vi "MinimalSynthApp.vi"(0 "Choose Directory":path) -> ()   [LabVIEW 2022 SP3]
uses:
  <vilib>/Analysis/NI_AALBase.lvlib
panel:
  out "Array":i16[][](array[numeric])
  out "x-y":u32
  in  "One Way Receive":bool
  in  "Recip processing":bool
  in  "Recip Processing":u16[][](array[ring])=[[1, 2, 2, 2, 2], [0, 1, 2, 2, 2], [0, 0, 1, 2, 2], [0, 0, 0, 1, 2], [0, 0, 0, 0, 1]] items=["0", "1", "2"]
  in  "Set to Focus":i32=1 min=1 max=5 step=1
  in  "Type of Mean":u16(ring)=3 items=["Mean from lines", "Mean just lines", "Poly Mean", "No mean"]
  in  "Display Plots":bool=TRUE
  in  "Axis scaling":bool=TRUE
  in  "Compress":bool
  in  "Tansducer":u16(ring)=1 items=["F2 40 MHz", "F3 20 MHz"]
  in  "F3 20 MHz":dbl[](array[numeric])=[0.0, 0.0021173000000000003, 0.002217038688303391, 0.003063649156506908, 0.0031631091439381287, 0.0038030513383040436, 0.003902223261134889, 0.004435332245982045, 0.004534208485358321, 0.004999044189180914]
  in  "Round to ROC?":bool=TRUE
  out "ROC (mm)":dbl=0.012
  out "Current File":string
  in  "file ext":string="*1to1*"
  out "zone size mm":dbl format="%#_3g"
  in  "Save Data":bool
  out "c (m/s)":i32=1485
  in  "F2 40MHz":sgl[](array[numeric])=[0.0, 0.00132, 0.00142, 0.0019, 0.002, 0.00236, 0.00245, 0.00275, 0.00285, 0.0031]
  in  "F- zones":i16=41
  out "Focal zones m":sgl[](array[numeric])=[0.0085, 0.009, 0.0095, 0.01, 0.0105, 0.011, 0.0115, 0.012, 0.0125, 0.013, 0.0135, 0.014, 0.0145, 0.015]
  out "Synth Aperture":dbl[][](graph)
  in  "Use Selected Files":bool
  in  "Listbox":i32[](listbox)
  # "Dimension of arrays for processing"
  # "XMT"
  # "RCV"
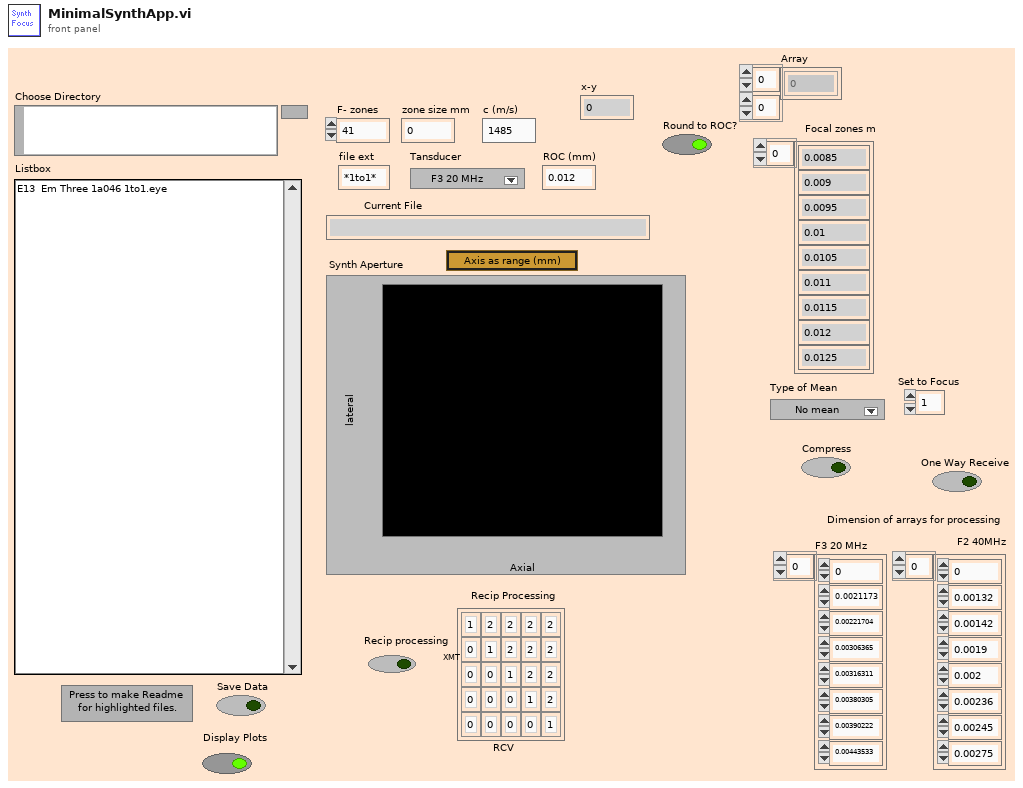
[diagram p1: front panel]
types:
  T1 = typedef "Header.ctl" = cluster{"header info":cluster{"Header":string, "Head length":i16}, "A/D info":cluster{"# rf points per line":u16, "# lines per scan":u16, "sample rate MHz":u16, "# A/D bits":i16, "# bytes per A/D":u16, "TGC Flag":u16, "A/D Type":string}, "Tranducer Info":cluster{"bandwidth":sgl, "center freq":sgl, "start freq":sgl, "ID":i32}, "Scan Info":cluster{"delay":sgl, "pivot distance":sgl, "sector scan angle":sgl, "operator":string, "Scan Mode":string, "location":string}, "Time/Date Info":cluster{"date":string, "time":string}, "RF Info":cluster{"RF file name":string, "RF file att":string, "RF cal file name":string, "RF cal file att":string}, "Patient Info":cluster{"ID":string, "extended ID":string, "age":u16, "sex":string, "previously\nscanned":string, "PSA":sgl, "LOS":u8, "Ethnicty 2":u8, "Race":u8}, "Tissue Type":cluster{"organ":i16, "disease type":i16, "disease location":i16}, "Votage scaling":cluster{"Digitizer (dB)":sgl, "Gain (dB)":sgl, "Atten (dB)":sgl}, "Comment":string, "Misc Info":cluster{"avg num":i16, "c speed":i16, "Div By or SF zones":i16, "XMIT CHS":u8, "RCV CHS":u8}, "Therapy Parameters":cluster{"Theraputic Freq (MHz)":sgl, "Time on (s)":sgl, "Therapy amplitude (mV)":sgl, "Lines Before":u16, "Lines After":u16}, "Scan Settings":cluster{"Energy (uJ or V)":u8, "Damp (Ohm) or Fc":u8, "HP Filt (KHz)":u8, "LP Filt (MHz)":u8, "Gain (db)":u8, "prf (kHz)":sgl, "Distance between\nscan lines (mm)":u16, "Distance between\nscan planes (mm)":u16}, "Compression Parameters":cluster{"F1 (MHz)":sgl, "F2 (MHz)":sgl, "% taper":sgl, "duration":sgl}, "Patient Info Xtra":cluster{"First Name":string, "Last Name":string, "Notes":string}}
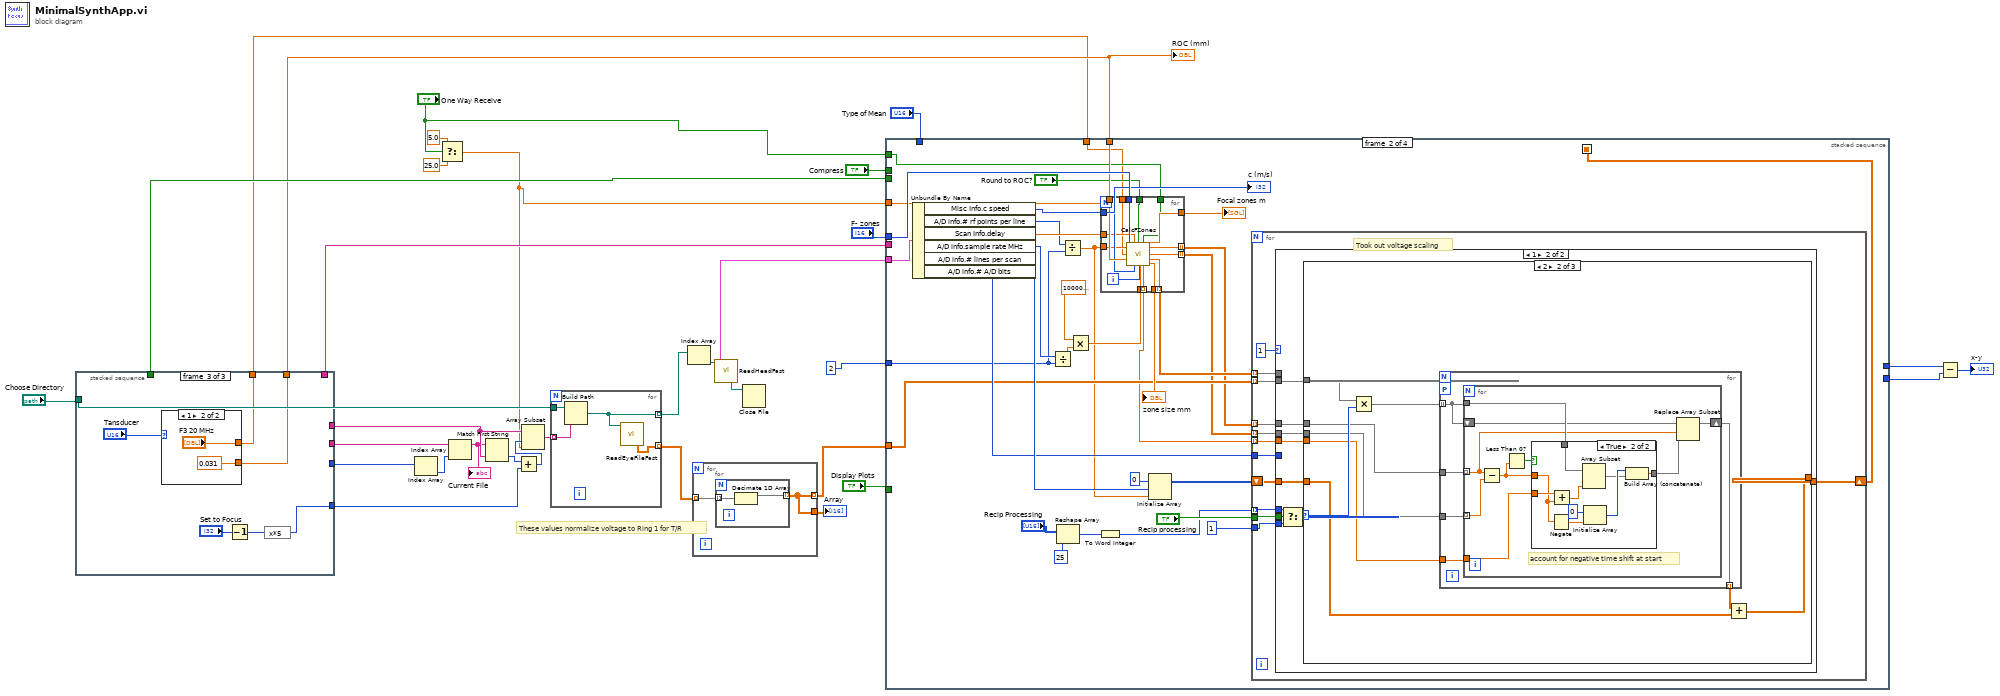
[diagram p0: block diagram]
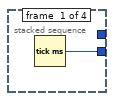
[diagram p2: hidden frame]
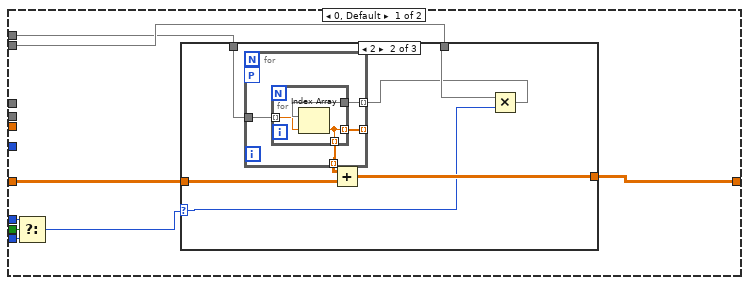
[diagram p3: hidden frame]
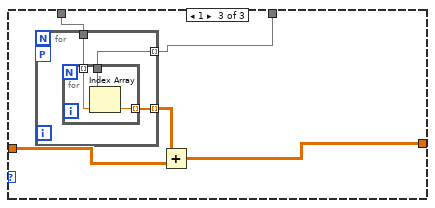
[diagram p5: hidden frame]
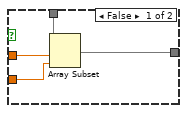
[diagram p7: hidden frame]
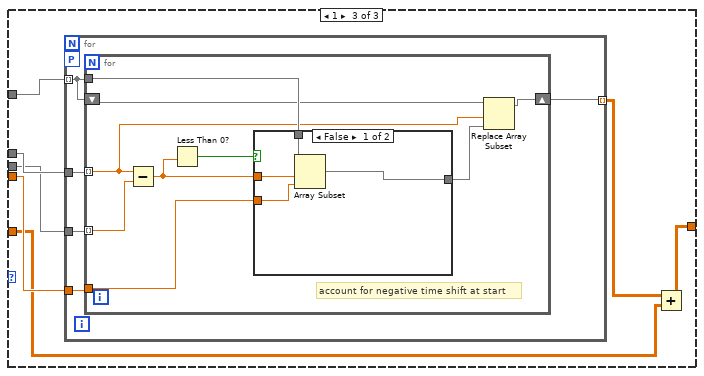
[diagram p8: hidden frame]
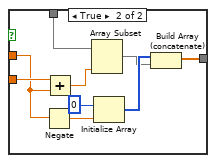
[diagram p9: hidden frame]
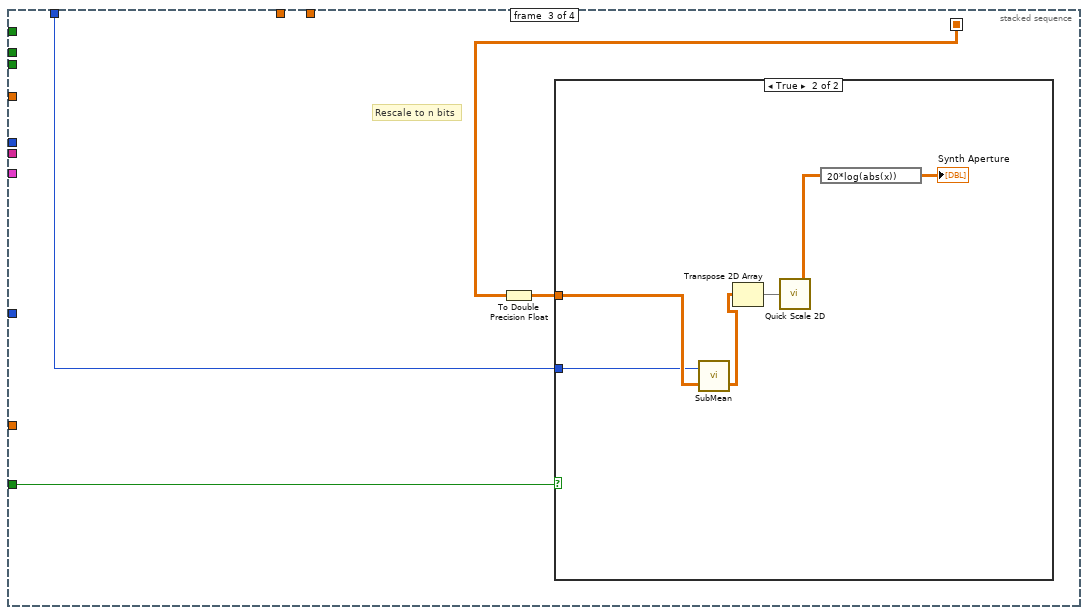
[diagram p10: hidden frame]
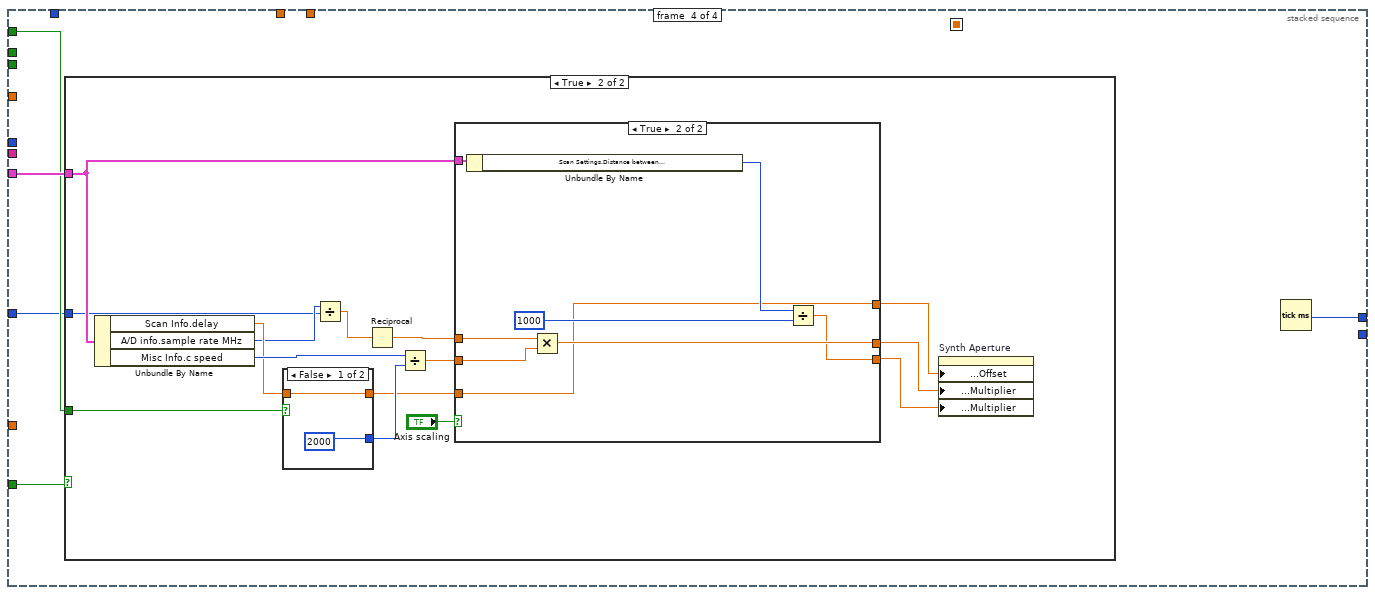
[diagram p12: hidden frame]
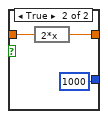
[diagram p14: hidden frame]
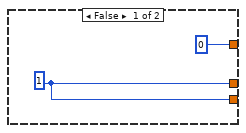
[diagram p15: hidden frame]
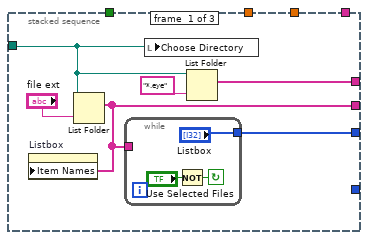
[diagram p16: hidden frame]
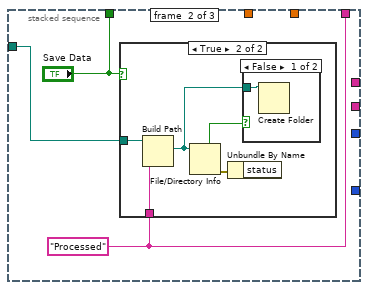
[diagram p17: hidden frame]
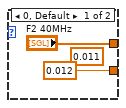
[diagram p20: hidden frame]
diagram:
  # "These values normalize voltage to Ring 1 for T/R"
  n1 = stacked-sequence {
    tunnel: "Choose Directory" -> [w37 w45 _]
    tunnel: [_ w43 _] -> w32
    tunnel: [_ "Save Data" _] -> w31
    tunnel: [w36 _ _] -> w30
    tunnel: [w35 _ _] -> w12
    tunnel: [w34 _ _] -> w29
    tunnel: [_ _ w56] -> w3
    tunnel: [_ _ w55] -> w28
    tunnel: [_ _ w52] -> w27
    frame #0 {
      n2 = List Folder(path=w37, pattern="file ext") -> (filenames=w34:string[])  [unwired: 1 in, 4 out]
      n3 = property on="Listbox" class="LstBox (strict)"("Item Names"=w34) -> ()  [unwired: 2 in, 2 out]
      n4 = while {
        tunnel: ["Listbox"] -> w35
        tunnel: w34 -> [_]
        stop <- w42 continue-if-true
        n5 = Not(x="Use Selected Files") -> (.not. x?=w42:bool)
      }
      n6 = local write "Choose Directory"(w37) -> ()
      n7 = List Folder(path=w37, pattern="*.eye" ("prompt")) -> (filenames=w36:string[])  [unwired: 1 in, 4 out]
    }
    frame #1 {
      w43 = "Processed"
      n8 = case shown="True" "Save Data" {
        tunnel: w45 -> [_ w49]
        tunnel: w43 -> [_ w47]
        frame False {
        }
        frame True {
          n9 = Build Path(base path=w49, name or relative path=w47) -> (appended path=w48:path)
          n10 = File/Directory Info(path=w48) -> (directory=w50:bool, error out=w46:errorcluster)  [unwired: 1 in, 5 out]
          n11 = Unbundle By Name(w46) -> ()  [unwired: 1 out]
          n12 = case shown="False" w50 {
            tunnel: w48 -> [w51 _]
            frame False {
              n13 = Create Folder(path (use dialog)=w51) -> ()  [unwired: 1 in, 4 out]
            }
            frame True {
            }
          }
        }
      }
    }
    frame #2 {
      n14 = case shown="1" "Tansducer" {
        tunnel: ["F2 40MHz" "F3 20 MHz"] -> w56
        tunnel: [0.012 ("ROC (mm)") 0.031 ("ROC (mm)")] -> w55
        frame 0, Default {
          (unwired) 0.011 ("ROC (mm)")
        }
        frame 1 {
        }
      }
      n15 = Decrement(x="Set to Focus") -> (x-1=w53:i32)
      n16 = expression code="x*5"(w53) -> (w52:i32)
    }
  }
  "ROC (mm)" <- w28
  n17 = Index Array(array=w12) -> (element=w11:i32)  [unwired: 1 in]
  n18 = Select(t=5.0, s="One Way Receive", f=25.0 ("t")) -> (s? t:f=w2:dbl)
  n19 = Index Array(array=w29, index=w11) -> (element=w22:string)
  "Current File" <- w22
  n20 = Match First String(2:w30, 3:w22) -> (0:w14:i32)  [unwired: 1 out]
  n21 = Add(x=w14, y=w27) -> (x+y=w13:i32)
  n22 = Array Subset(array=w30, index=w13, length=w2) -> (w23:string[])
  n23 = for {
    tunnel: "Choose Directory" -> [w65]
    tunnel: w23 -> [w64] mode=indexing
    tunnel: [w63] -> w18 mode=indexing
    tunnel: [w62] -> w5 mode=indexing
    n24 = Build Path(base path=w65, name or relative path=w64) -> (appended path=w63:path)
    n25 = call "ReadEyeFileFast.vi"("new file path"=w63) -> ("2-D data array"=w62:sgl[][])  [unwired: 1 in, 17 out]
  }
  n26 = Index Array(array=w18) -> (element=w19:path)  [unwired: 1 in]
  n27 = for {
    tunnel: w5 -> [w67] mode=indexing
    tunnel: [w66] -> w4 mode=indexing
    tunnel: [w66] -> w1
    n28 = for {
      tunnel: w67 -> [w69] mode=indexing
      tunnel: [w68] -> w66 mode=indexing
      n29 = Decimate 1D Array(w69) -> (w68:sgl[])  [unwired: 1 out]
    }
  }
  "Array" <- w1
  n30 = call "ReadHeadFast.vi"("new file path"=w19) -> ("Header In"=w20:T1, "refnum out"=w15:refnum<file>)  [unwired: 2 in, 15 out]
  n31 = Close File(refnum=w15) -> ()  [unwired: 1 in, 2 out]
  n32 = stacked-sequence {
    seq-local: [_ w99 _ _] -> [_ _ w250 _]
    tunnel: w20 -> [_ w102 _ w262]
    tunnel: "F- zones" -> [_ w101 _ _]
    tunnel: w31 -> [_ _ _ _]
    tunnel: w32 -> [_ _ _ _]
    tunnel: w28 -> [_ w94 _ _]
    tunnel: "Compress" -> [_ _ _ _]
    tunnel: "Display Plots" -> [_ _ w251 w261]
    tunnel: "Type of Mean" -> [_ _ w249 _]
    tunnel: "One Way Receive" -> [_ w88 _ w260]
    tunnel: w4 -> [_ w86 _ _]
    tunnel: [w70 _ _ _] -> w8
    tunnel: [_ _ _ w258] -> w9
    tunnel: 2 -> [_ w78 _ w259]
    tunnel: w3 -> [_ w72 _ _]
    tunnel: w2 -> [_ w71 _ _]
    frame #0 {
      n33 = Tick Count (ms)() -> (millisecond timer value=w70:u32)
    }
    frame #1 {
      n34 = Unbundle By Name(w102) -> ("Misc Info.c speed"=w93:i16, "A/D info.# rf points per line"=w79:u16, "Scan Info.delay"=w85:sgl, "A/D info.sample rate MHz"=w82:u16, "A/D info.# lines per scan"=w98:u16, "A/D info.# A/D bits"=w97:i16)
      "c (m/s)" <- w93
      n35 = Divide(x=w82, y=w78) -> (x/y=w81:dbl)
      n36 = Reshape Array("Recip Processing", 25) -> (w91:u16[])
      n37 = Divide(x=w79, y=w78) -> (x/y=w80:dbl)
      n38 = Multiply(x=1000000.0, y=w81) -> (x*y=w96:dbl)
      n39 = To Word Integer(number=w91) -> (16bit integer=w77:i16[])
      n40 = for {
        N: w71 -> [_]
        tunnel: w101 -> [w120]
        tunnel: [w119] -> w100
        tunnel: w96 -> [w118]
        tunnel: [w117] -> w95
        tunnel: w94 -> [w116]
        tunnel: w93 -> [w115]
        tunnel: "Round to ROC?" -> [w114]
        tunnel: w88 -> [w113]
        tunnel: w85 -> [w112]
        tunnel: w80 -> [w111]
        tunnel: [w110] -> w76 mode=indexing
        tunnel: [w109] -> w75 mode=indexing
        tunnel: [w108] -> w74 mode=indexing
        tunnel: [w107] -> w73 mode=indexing
        tunnel: w72 -> [w106]
        i -> [w105]
        n41 = call "CalcFZones.vi"("F- zones"=w120, "delay (mm)"=w112, "Round to ROC?"=w114, "One Way Receive"=w113, "# rf points per line"=w111, "Radii (m)"=w106, "ROC (m)"=w116, "Sampling Rate"=w118, "c (m/s)"=w115, "File index number"=w105) -> ("FZones (m)"=w117:dbl[], "ZoneStart"=w109:sgl[], "ZoneShift"=w108:sgl[], "ZoneLength"=w110:sgl[], "zone size mm"=w107:dbl, "IndexVals"=w119:sgl[])
      }
      "Focal zones m" <- w95
      "zone size mm" <- w100
      n42 = Initialize Array(i16 0, w98, w80) -> (w90:i16[][])
      n43 = for {
        shift-right: [w130] -> w99
        shift-left: w90 -> [w131]
        tunnel: w97 -> [w132]
        tunnel: w77 -> [w128] mode=indexing
        tunnel: w86 -> [w126] mode=indexing
        tunnel: "Recip processing" -> [w129]
        tunnel: i16 1 -> [w127]
        tunnel: w76 -> [w125] mode=indexing
        tunnel: w75 -> [w124] mode=indexing
        tunnel: w74 -> [w123] mode=indexing
        tunnel: w73 -> [w122] mode=indexing
        # "Took out voltage scaling"
        n44 = case shown="1" 1 {
          tunnel: w132 -> [_ _]
          tunnel: w131 -> [w140 w176]
          tunnel: [w139 w175] -> w130
          tunnel: w129 -> [w138 w174]
          tunnel: w128 -> [w137 w173]
          tunnel: w127 -> [w135 w171]
          tunnel: w126 -> [w134 w170]
          tunnel: w125 -> [w133 _]
          tunnel: w124 -> [_ w169]
          tunnel: w123 -> [_ w168]
          tunnel: w122 -> [_ w167]
          frame 0, Default {
            n45 = Select(t=w137, s=w138, f=w135) -> (s? t:f=w136:i16)
            n46 = case shown="2" w136 {
              selector: w136 -> [_ w145 _]
              tunnel: [w141 w147 w159] -> w139
              tunnel: w134 -> [_ w146 w158]
              tunnel: w140 -> [w141 w148 w160]
              tunnel: w133 -> [_ w142 w156]
              frame 0, Default {
              }
              frame 2 {
                n47 = Multiply(x=w146, y=w145) -> (x*y=w144:sgl[][])
                n48 = for {
                  tunnel: [w152] -> _ mode=indexing
                  workers-P: _ -> [_]
                  tunnel: w144 -> [w151] mode=indexing
                  tunnel: [w150] -> w143 mode=indexing
                  tunnel: w142 -> [w149]
                  n49 = for {
                    tunnel: [w154] -> w152 mode=indexing
                    tunnel: w151 -> [w155]
                    tunnel: [w154] -> w150 mode=indexing
                    tunnel: w149 -> [w153] mode=indexing
                    n50 = Index Array(array=w155, index=w153) -> (element=w154:sgl)
                  }
                }
                n51 = Add(x=w143, y=w148) -> (x+y=w147:sgl[][])
              }
              frame 1 {
                n52 = for {
                  tunnel: [w163] -> w157 mode=indexing
                  workers-P: _ -> [_]
                  tunnel: w158 -> [w162] mode=indexing
                  tunnel: w156 -> [w161]
                  n53 = for {
                    tunnel: [w166] -> w163 mode=indexing
                    tunnel: w162 -> [w165]
                    tunnel: w161 -> [w164] mode=indexing
                    n54 = Index Array(array=w165, index=w164) -> (element=w166:sgl)
                  }
                }
                n55 = Add(x=w157, y=w160) -> (x+y=w159:sgl[][])
              }
            }
          }
          frame 1 {
            n56 = Select(t=w173, s=w174, f=w171) -> (s? t:f=w172:i16)
            n57 = case shown="2" w172 {
              selector: w172 -> [_ w185 _]
              tunnel: [w177 w179 w216] -> w175
              tunnel: w170 -> [_ w186 w220]
              tunnel: w176 -> [w177 w178 w214]
              tunnel: w169 -> [_ w183 w219]
              tunnel: w168 -> [_ w182 w218]
              tunnel: w167 -> [_ w181 w217]
              frame 0, Default {
              }
              frame 2 {
                n58 = Multiply(x=w186, y=w185) -> (x*y=w184:sgl[][])
                n59 = for {
                  tunnel: w184 -> [w191] mode=indexing
                  tunnel: w183 -> [w190]
                  tunnel: w182 -> [w189]
                  tunnel: w181 -> [w188]
                  workers-P: _ -> [_]
                  tunnel: [w187] -> w180 mode=indexing
                  n60 = for {
                    tunnel: w190 -> [w193] mode=indexing
                    tunnel: w188 -> [w200]
                    tunnel: w189 -> [w199] mode=indexing
                    tunnel: w191 -> [w196]
                    shift-right: [w195] -> w187
                    shift-left: w191 -> [w194]
                    # "account for negative time shift at start"
                    n61 = Subtract(x=w193, y=w199) -> (x-y=w197:sgl)
                    n62 = Less Than 0?(x=w197) -> (x < 0?=w198:bool)
                    n63 = case shown="True" w198 {
                      tunnel: w196 -> [w204 w212]
                      tunnel: w200 -> [w202 w213]
                      tunnel: [w203 w207] -> w192
                      tunnel: w197 -> [w201 w210]
                      frame False {
                        n64 = Array Subset(array=w204, index=w201, length=w202) -> (w203:sgl[])
                      }
                      frame True {
                        n65 = Negate(x=w210) -> (-x=w205:sgl)
                        n66 = Add(x=w213, y=w210) -> (x+y=w206:dbl)
                        n67 = Array Subset(array=w212, length=w206) -> (w208:sgl[])  [unwired: 1 in]
                        n68 = Initialize Array(i16 0, w205) -> (w209:i16[])
                        n69 = Build Array (concatenate)(w209, w208) -> (w207:sgl[])
                      }
                    }
                    n70 = Replace Array Subset(array=w194, new element=w192, index=w193) -> (w195:sgl[])
                  }
                }
                n71 = Add(x=w180, y=w178) -> (x+y=w179:sgl[][])
              }
              frame 1 {
                n72 = for {
                  tunnel: w220 -> [w225] mode=indexing
                  tunnel: w219 -> [w224]
                  tunnel: w218 -> [w223]
                  tunnel: w217 -> [w222]
                  tunnel: [w221] -> w215 mode=indexing
                  workers-P: _ -> [_]
                  n73 = for {
                    tunnel: w224 -> [w227] mode=indexing
                    tunnel: w222 -> [w234]
                    tunnel: w223 -> [w233] mode=indexing
                    tunnel: w225 -> [w230]
                    shift-right: [w229] -> w221
                    shift-left: w225 -> [w228]
                    # "account for negative time shift at start"
                    n74 = Subtract(x=w227, y=w233) -> (x-y=w231:sgl)
                    n75 = Less Than 0?(x=w231) -> (x < 0?=w232:bool)
                    n76 = case shown="False" w232 {
                      tunnel: w230 -> [w238 w246]
                      tunnel: w234 -> [w236 w247]
                      tunnel: [w237 w241] -> w226
                      tunnel: w231 -> [w235 w244]
                      frame False {
                        n77 = Array Subset(array=w238, index=w235, length=w236) -> (w237:sgl[])
                      }
                      frame True {
                        n78 = Negate(x=w244) -> (-x=w239:sgl)
                        n79 = Add(x=w247, y=w244) -> (x+y=w240:dbl)
                        n80 = Array Subset(array=w246, length=w240) -> (w242:sgl[])  [unwired: 1 in]
                        n81 = Initialize Array(i16 0, w239) -> (w243:i16[])
                        n82 = Build Array (concatenate)(w243, w242) -> (w241:sgl[])
                      }
                    }
                    n83 = Replace Array Subset(array=w228, new element=w226, index=w227) -> (w229:sgl[])
                  }
                }
                n84 = Add(x=w215, y=w214) -> (x+y=w216:sgl[][])
              }
            }
          }
        }
      }
    }
    frame #2 {
      # "Rescale to n bits"
      n85 = To Double Precision Float(number=w250) -> (double precision float=w248:dbl[][])
      n86 = case shown="True" w251 {
        tunnel: w248 -> [_ w254]
        tunnel: w249 -> [_ w252]
        frame False {
        }
        frame True {
          n87 = call "SubMean.vi"("Scan Data In"=w254, "Type of Mean"=w252) -> ("Array"=w253:dbl[][])  [unwired: 1 out]
          n88 = Transpose 2D Array(2D array=w253) -> (transposed array=w257:dbl[][])
          n89 = call <vilib>:"Quick Scale 2D.vi"("X"=w257) -> ("Yij=Xij/Max|X|"=w256:dbl[][])  [unwired: 2 out]
          n90 = expression code="20*log(abs(x))"(w256) -> (→"Synth Aperture":dbl[][])
        }
      }
    }
    frame #3 {
      n91 = case shown="True" w261 {
        tunnel: w262 -> [_ w274]
        tunnel: w260 -> [_ w269]
        tunnel: w259 -> [_ w263]
        frame False {
        }
        frame True {
          n92 = Unbundle By Name(w274) -> ("Scan Info.delay"=w267:sgl, "A/D info.sample rate MHz"=w264:u16, "Misc Info.c speed"=w276:i16)
          n93 = case shown="False" w269 {
            tunnel: [2000 1000] -> w268
            tunnel: w267 -> [w278 w281]
            tunnel: [w278 w280] -> w266
            frame False {
            }
            frame True {
              n94 = expression code="2*x"(w281) -> (w280:sgl)
            }
          }
          n95 = Divide(x=w264, y=w263) -> (x/y=w265:dbl)
          n96 = Reciprocal(x=w265) -> (1/x=w277:dbl)
          n97 = Divide(x=w276, y=w268) -> (x/y=w275:dbl)
          n98 = case shown="True" "Axis scaling" {
            tunnel: [w284 w291] -> w270
            tunnel: w277 -> [_ w292]
            tunnel: w274 -> [_ w290]
            tunnel: [w284 w287] -> w272
            tunnel: [0 w285] -> w271
            tunnel: w275 -> [_ w286]
            tunnel: w266 -> [_ w285]
            frame False {
              w284 = 1
            }
            frame True {
              n99 = Unbundle By Name(w290) -> ("Scan Settings.Distance between\nscan lines (mm)"=w289:u16)
              n100 = Multiply(x=w292, y=w286) -> (x*y=w291:dbl)
              n101 = Divide(x=w289, y=1000) -> (x/y=w287:dbl)
            }
          }
          n102 = property on="Synth Aperture" class="IntGraph (strict)"("X Scale.Offset and Multiplier:Offset"=w271, "X Scale.Offset and Multiplier:Multiplier"=w270, "Y Scale.Offset and Multiplier:Multiplier"=w272) -> ()  [unwired: 2 in, 2 out]
        }
      }
      n103 = Tick Count (ms)() -> (millisecond timer value=w258:u32)
    }
  }
  n104 = Subtract(x=w9, y=w8) -> (x-y=→"x-y":u32)
